vi "S4GUI_003.vi"(7 "Tab ObsEng":enum32{"Obs", "CCD modes", "Guider", "Eng"}(tab)) -> ()   [LabVIEW 2018] (continued)
        n5068 = call "Read ASEL.vi"("error in (no error)"=w12170, "Instrument in"=w12171) -> ("error out"=w12167:errorcluster, "Opt_Selector.lvclass"=w12169:refnum<class "Opt_Selector.lvclass">, "Instrument out"=w12165:refnum<class "Instrument.lvclass">)  [unwired: 7 in]
        n5069 = call "Write target.vi"("error in (no error)"=w12167, "target"=w12168, "Optics in"=w12169) -> ("error out"=w12164:errorcluster, "Optics out"=w12166:refnum<class "Opt_Selector.lvclass">)  [unwired: 7 in]
        n5070 = call "Write ASEL.vi"("error in (no error)"=w12164, "Opt_Selector.lvclass"=w12166, "Instrument in"=w12165) -> ("error out"=w12161:errorcluster, "Instrument out"=w12163:refnum<class "Instrument.lvclass">)  [unwired: 7 in]
        n5071 = call "Write Instrument.lvclass.vi"("error in (no error)"=w12161, "Instrument.lvclass"=w12163, "S4ACS_GUI in"=w12162) -> ("error out"=w12160:errorcluster, "S4ACS_GUI out"=w12159:refnum<class "S4GUI.lvclass">)  [unwired: 7 in]
      }
      event "ASEL_set": Value Change {
        n5072 = event-data() -> ()  [unwired: 1 in, 4 out]
        n5073 = call "Read Instrument.lvclass.vi"("error in (no error)"=w12192, "S4ACS_GUI in"=w12193) -> ("error out"=w12190:errorcluster, "Instrument.lvclass"=w12191:refnum<class "Instrument.lvclass">, "S4ACS_GUI out"=w12178:refnum<class "S4GUI.lvclass">)  [unwired: 7 in]
        n5074 = call "Read ASEL.vi"("error in (no error)"=w12190, "Instrument in"=w12191) -> ("error out"=w12187:errorcluster, "Opt_Selector.lvclass"=w12189:refnum<class "Opt_Selector.lvclass">, "Instrument out"=w12181:refnum<class "Instrument.lvclass">)  [unwired: 7 in]
        n5075 = call-dynamic "Read State Machine.vi"("error in (no error)"=w12187, "Device in"=w12189) -> ("error out"=w12186:errorcluster, "State Machine.lvclass"=w12175:refnum<class "State Machine.lvclass">, "Device out"=w12183:refnum<class "Opt_Selector.lvclass">)  [unwired: 7 in]
        n5076 = call "Next State.vi"("error in (no error)"=w12186, "New_State"=1, "State Machine in"=w12175) -> ("error out"=w12185:errorcluster, "State Machine out"=w12184:refnum<class "State Machine.lvclass">)  [unwired: 7 in]
        n5077 = call-dynamic "Write State Machine.vi"("error in (no error)"=w12185, "State Machine.lvclass"=w12184, "Device in"=w12183) -> ("error out"=w12180:errorcluster, "Device out"=w12182:refnum<class "Opt_Selector.lvclass">)  [unwired: 7 in]
        n5078 = call "Write ASEL.vi"("error in (no error)"=w12180, "Opt_Selector.lvclass"=w12182, "Instrument in"=w12181) -> ("error out"=w12177:errorcluster, "Instrument out"=w12179:refnum<class "Instrument.lvclass">)  [unwired: 7 in]
        n5079 = call "Write Instrument.lvclass.vi"("error in (no error)"=w12177, "Instrument.lvclass"=w12179, "S4ACS_GUI in"=w12178) -> ("error out"=w12176:errorcluster, "S4ACS_GUI out"=w12174:refnum<class "S4GUI.lvclass">)  [unwired: 7 in]
      }
      event "ASEL_stop": Value Change {
        n5080 = event-data() -> ()  [unwired: 1 in, 4 out]
        n5081 = call "Read Instrument.lvclass.vi"("error in (no error)"=w12212, "S4ACS_GUI in"=w12213) -> ("error out"=w12210:errorcluster, "Instrument.lvclass"=w12211:refnum<class "Instrument.lvclass">, "S4ACS_GUI out"=w12197:refnum<class "S4GUI.lvclass">)  [unwired: 7 in]
        n5082 = call "Read ASEL.vi"("error in (no error)"=w12210, "Instrument in"=w12211) -> ("error out"=w12206:errorcluster, "Opt_Selector.lvclass"=w12209:refnum<class "Opt_Selector.lvclass">, "Instrument out"=w12200:refnum<class "Instrument.lvclass">)  [unwired: 7 in]
        n5083 = call-dynamic "Read State Machine.vi"("error in (no error)"=w12206, "Device in"=w12209) -> ("error out"=w12205:errorcluster, "State Machine.lvclass"=w12208:refnum<class "State Machine.lvclass">, "Device out"=w12202:refnum<class "Opt_Selector.lvclass">)  [unwired: 7 in]
        n5084 = call "Next State.vi"("error in (no error)"=w12205, "New_State"=10, "State Machine in"=w12208) -> ("error out"=w12204:errorcluster, "State Machine out"=w12203:refnum<class "State Machine.lvclass">)  [unwired: 7 in]
        n5085 = call-dynamic "Write State Machine.vi"("error in (no error)"=w12204, "State Machine.lvclass"=w12203, "Device in"=w12202) -> ("error out"=w12199:errorcluster, "Device out"=w12201:refnum<class "Opt_Selector.lvclass">)  [unwired: 7 in]
        n5086 = call "Write ASEL.vi"("error in (no error)"=w12199, "Opt_Selector.lvclass"=w12201, "Instrument in"=w12200) -> ("error out"=w12196:errorcluster, "Instrument out"=w12198:refnum<class "Instrument.lvclass">)  [unwired: 7 in]
        n5087 = call "Write Instrument.lvclass.vi"("error in (no error)"=w12196, "Instrument.lvclass"=w12198, "S4ACS_GUI in"=w12197) -> ("error out"=w12195:errorcluster, "S4ACS_GUI out"=w12194:refnum<class "S4GUI.lvclass">)  [unwired: 7 in]
      }
      event "ASEL_init": Value Change {
        n5088 = event-data() -> ()  [unwired: 1 in, 4 out]
        n5089 = call "Read Instrument.lvclass.vi"("error in (no error)"=w12232, "S4ACS_GUI in"=w12233) -> ("error out"=w12230:errorcluster, "Instrument.lvclass"=w12231:refnum<class "Instrument.lvclass">, "S4ACS_GUI out"=w12217:refnum<class "S4GUI.lvclass">)  [unwired: 7 in]
        n5090 = call "Read ASEL.vi"("error in (no error)"=w12230, "Instrument in"=w12231) -> ("error out"=w12226:errorcluster, "Opt_Selector.lvclass"=w12229:refnum<class "Opt_Selector.lvclass">, "Instrument out"=w12220:refnum<class "Instrument.lvclass">)  [unwired: 7 in]
        n5091 = call-dynamic "Read State Machine.vi"("error in (no error)"=w12226, "Device in"=w12229) -> ("error out"=w12225:errorcluster, "State Machine.lvclass"=w12228:refnum<class "State Machine.lvclass">, "Device out"=w12222:refnum<class "Opt_Selector.lvclass">)  [unwired: 7 in]
        n5092 = call "Next State.vi"("error in (no error)"=w12225, "New_State"=30, "State Machine in"=w12228) -> ("error out"=w12224:errorcluster, "State Machine out"=w12223:refnum<class "State Machine.lvclass">)  [unwired: 7 in]
        n5093 = call-dynamic "Write State Machine.vi"("error in (no error)"=w12224, "State Machine.lvclass"=w12223, "Device in"=w12222) -> ("error out"=w12219:errorcluster, "Device out"=w12221:refnum<class "Opt_Selector.lvclass">)  [unwired: 7 in]
        n5094 = call "Write ASEL.vi"("error in (no error)"=w12219, "Opt_Selector.lvclass"=w12221, "Instrument in"=w12220) -> ("error out"=w12216:errorcluster, "Instrument out"=w12218:refnum<class "Instrument.lvclass">)  [unwired: 7 in]
        n5095 = call "Write Instrument.lvclass.vi"("error in (no error)"=w12216, "Instrument.lvclass"=w12218, "S4ACS_GUI in"=w12217) -> ("error out"=w12215:errorcluster, "S4ACS_GUI out"=w12214:refnum<class "S4GUI.lvclass">)  [unwired: 7 in]
      }
    }
    n5096 = Unbundle By Name(w122) -> ("status"=w121:bool)
    n5097 = flat-sequence {
      tunnel: w136 -> [w151]
      tunnel: w134 -> [w149]
      tunnel: [w151] -> w133
      tunnel: [w147] -> w132
      tunnel: [w146] -> w131
      tunnel: [w154] -> w135
      tunnel: w133 -> [w154]
      tunnel: w132 -> [w153]
      tunnel: w131 -> [w152]
      frame #0 {
        n5098 = Tick Count (ms)() -> (millisecond timer value=w150:u32)
        n5099 = local read "loop max(ms)"() -> (w145:u32)
        n5100 = Subtract(x=w150, y=w149) -> (x-y=w147:u32)
        n5101 = Greater?(x=w147, y=w145) -> (0:w148:bool)
        n5102 = Select(t=w147, s=w148, f=w145) -> (s? t:f=w146:u32)
      }
      frame #1 {
        "loop time(ms)" <- w153
        "loop max(ms)" <- w152
      }
    }
    n5103 = Or(x=w121, y=w120) -> (x .or. y?=w119:bool)
  }
  "error out 9" <- w2
  n5104 = while {
    tunnel: w9 -> [_]
    stop <- FALSE stop-if-true
    n5105 = disable-structure shown="Enabled" {
      frame Disabled {
        n5106 = call "ZeroMQ_ACS1.vi"() -> ()  [unwired: 12 in]
        n5107 = call "ZeroMQ_ACS2.vi"() -> ()  [unwired: 12 in]
        n5108 = call "ZeroMQ_ACS3.vi"() -> ()  [unwired: 12 in]
        n5109 = call "ZeroMQ_ACS4.vi"() -> ()  [unwired: 12 in]
        n5110 = disable-structure shown="Enabled" {
          frame Disabled {
            n5111 = call "ZeroMQ_FOC.vi"() -> ()  [unwired: 12 in]
          }
          frame Enabled {
            n5112 = call "ZeroMQ_FOC_REQREP.vi"() -> ()  [unwired: 12 in]
          }
        }
        n5113 = call "ZeroMQ_WSTA.vi"() -> ()  [unwired: 12 in]
        n5114 = call "ZeroMQ_TCS.vi"() -> ()  [unwired: 12 in]
        n5115 = call "ZeroMQ_S4ICS.vi"() -> ()  [unwired: 12 in]
        n5116 = call "ZeroMQ_SUBGS.vi"() -> ()  [unwired: 12 in]
        n5117 = call "StreamTransmitSyncBox.vi"() -> ()  [unwired: 12 in]
        n5118 = call "StreamReceiveSyncBox.vi"() -> ()  [unwired: 12 in]
        n5119 = call "ZeroMQ_PUB.vi"() -> ()  [unwired: 12 in]
      }
      frame Enabled {
        n5120 = call "communication manager.vi"() -> ()  [unwired: 12 in]
      }
    }
  }
  n5121 = stacked-sequence "INTERFACE" {
    frame #0 {
    }
    frame #1 {
    }
    frame #2 {
    }
    frame #3 {
    }
    frame #4 {
    }
  }
  n5122 = call-dynamic "Log Error.vi"("error in (no error)"=w2, "S4GUI in"=w4) -> ("error out"=→"error out 10":errorcluster, "S4GUI out"=w3:refnum<class "S4GUI.lvclass">)  [unwired: 8 in]
  n5123 = call-dynamic "End.vi"("S4ACS_GUI in"=w3) -> ("error out"=w21:errorcluster)  [unwired: 9 in, 1 out]
  n5124 = flat-sequence {
    tunnel: [w12236] -> w19
    tunnel: w21 -> [w12238]
    tunnel: [w12244] -> w20
    tunnel: w19 -> [w12244]
    frame #0 {
      w12242 = FALSE
      # "Apaga todos os leds, habilita Tab ObsEng."
      n5125 = property on="Tab ObsEng" class="TabCtl (strict)"("Tabs Visible?"=TRUE) -> ()  [unwired: 2 in, 2 out]
      n5126 = property on="Channel 4" class="Bool (strict)"("Value"=w12242) -> ()  [unwired: 2 in, 2 out]
      n5127 = property on="Channel 3" class="Bool (strict)"("Value"=w12242) -> ()  [unwired: 2 in, 2 out]
      n5128 = property on="Channel 2" class="Bool (strict)"("Value"=w12242) -> ()  [unwired: 2 in, 2 out]
      n5129 = property on="Channel 1" class="Bool (strict)"("Value"=w12242) -> ()  [unwired: 2 in, 2 out]
      n5130 = property on="S4ICSoft" class="Bool (strict)"("Value"=w12242) -> ()  [unwired: 2 in, 2 out]
      n5131 = call <vilib>:"Clear Errors.vi"("error in (no error)"=w12238) -> ("error out"=w12235:errorcluster)  [unwired: 5 in, 1 out]
      n5132 = property on="TCSPD" class="Bool (strict)"("Value"=w12242) -> ()  [unwired: 2 in, 2 out]
      n5133 = property on="Focus 160" class="Bool (strict)"("Value"=w12242) -> ()  [unwired: 2 in, 2 out]
      n5134 = property on="Weather" class="Bool (strict)"("Value"=w12242) -> ()  [unwired: 2 in, 2 out]
      n5135 = property on="GUIDER" class="Bool (strict)"("Value"=w12242) -> ()  [unwired: 2 in, 2 out]
      n5136 = disable-structure shown="Disabled" {
        frame Disabled {
          n5137 = local write "Last Error"("" ("Last Error")) -> ()
        }
        frame Enabled {
        }
      }
      n5138 = property on="Last Error" class="Str"(error in=w12235, "Text.BG Color"=u32 13816530 ("Color Box"), "Caption.FontBold"=FALSE ("Caption.Font:Bold")) -> (error out=w12237:errorcluster)  [unwired: 1 in, 1 out]
      n5139 = call <vilib>:"Clear Errors.vi"("error in (no error)"=w12237) -> ("error out"=w12236:errorcluster)  [unwired: 5 in, 1 out]
    }
    frame #1 {
      n5140 = Stop() -> ()  [unwired: 1 in]
    }
  }
  "error out" <- w20
  "GUI version" <- w22
